vi "Item.vi"(8 "error in (no error)":errorcluster, 10 "Key":string, 11 "Map in":refnum<class "ObjectMap.lvclass">) -> (0 "error out":errorcluster, 1 "Value":refnum<class>, 3 "Map out":refnum<class "ObjectMap.lvclass">)   [LabVIEW 2013, in "LapDog.Collections.v_.Maps.lvlib" / "ObjectMap.lvclass"]
doc: "Returns a copy of the value associated with the given key.\n\nIf the key does not exist, error 510203 is returned."
uses:
  ObjectMap.lvclass
  MapImp/MapImp.lvclass
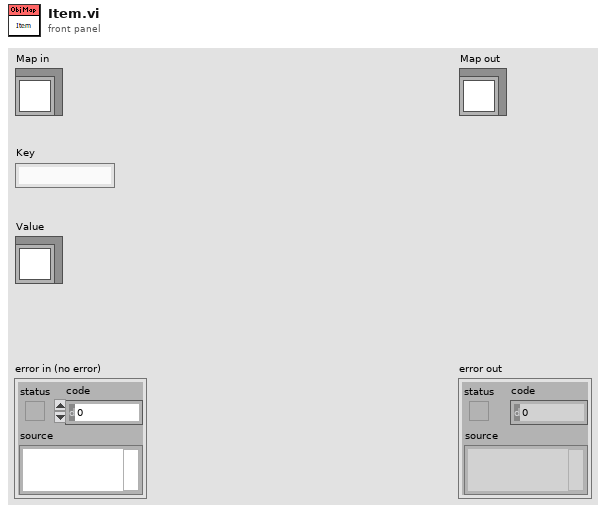
[diagram p1: front panel]
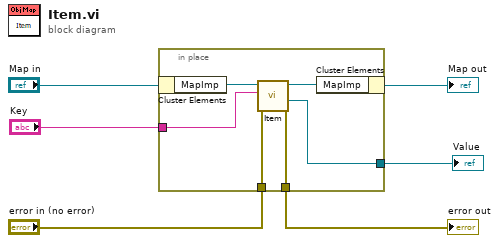
[diagram p0: block diagram]
diagram:
  n1 = in-place {
    in-place-border: "error in (no error)" -> [w10]
    in-place-border: [w9] -> w3
    in-place-border: "Key" -> [w8]
    in-place-border: [w7] -> w1
    n2 = in-place-cluster #1("Map in") -> ("MapImp"=w12:refnum<class "MapImp.lvclass">)
    n3 = call-dynamic "Item.vi"("error in (no error)"=w10, "Key"=w8, "VariantAttribute in"=w12) -> ("error out"=w9:errorcluster, "Value"=w7:refnum<class>, "VariantAttribute out"=w11:refnum<class "MapImp.lvclass">)  [unwired: 6 in]
    n4 = in-place-cluster #1("MapImp"=w11) -> (→"Map out":refnum<class "ObjectMap.lvclass">)
  }
  "error out" <- w3
  "Value" <- w1
